vi "sutter_control2.vi"() -> ()   [LabVIEW 2014]
uses:
  <vilib>/Instr/_visa.llb/VISA Configure Serial Port (Instr).vi
panel:
  in  "下拉列表":u16(ring) items=["M1"=1, "M2"=2, "M3"=3, "M4"=4]
  in  "error in (no error)":errorcluster
  in  "Go Home":bool
  in  "stop":bool
  out "error out":errorcluster
  out "z-position":dbl
  out "y-position":dbl
  out "x-position":dbl
  in  "Z um":dbl
  in  "Y um":dbl
  in  "X um":dbl
  in  "VISA resource name":refnum<visa-resource-name>
  # "Back to (0 0 0)"
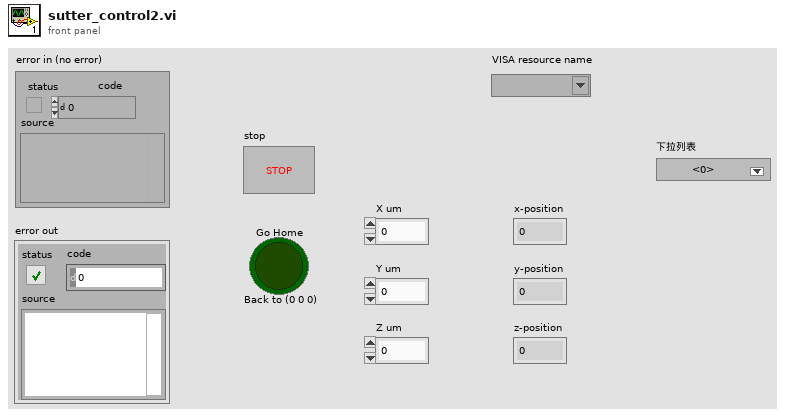
[diagram p1: front panel]
types:
  T1 = cluster{"Motor":u16, "X Pos":dbl, "Y Pos":dbl, "Z Pos":dbl, "Go Home":bool}
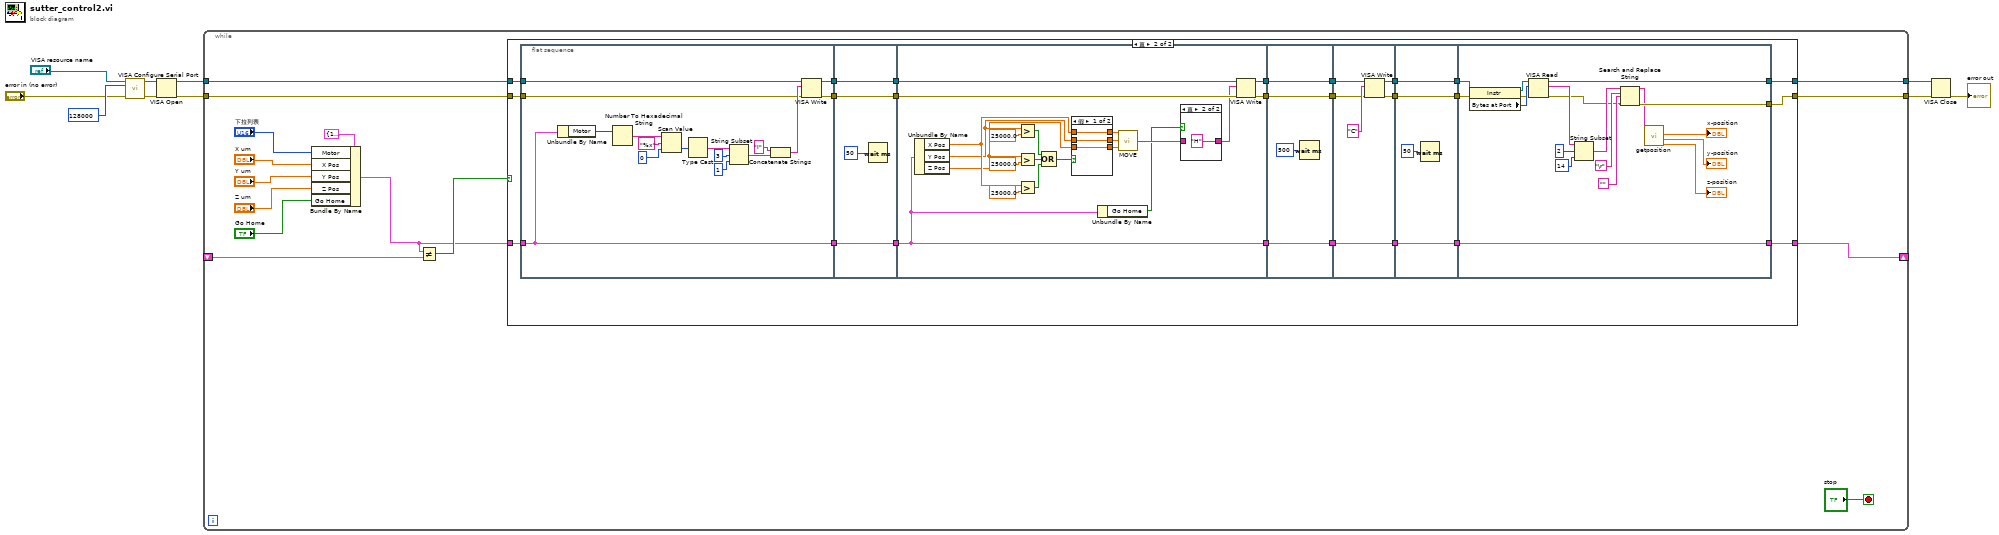
[diagram p0: block diagram]
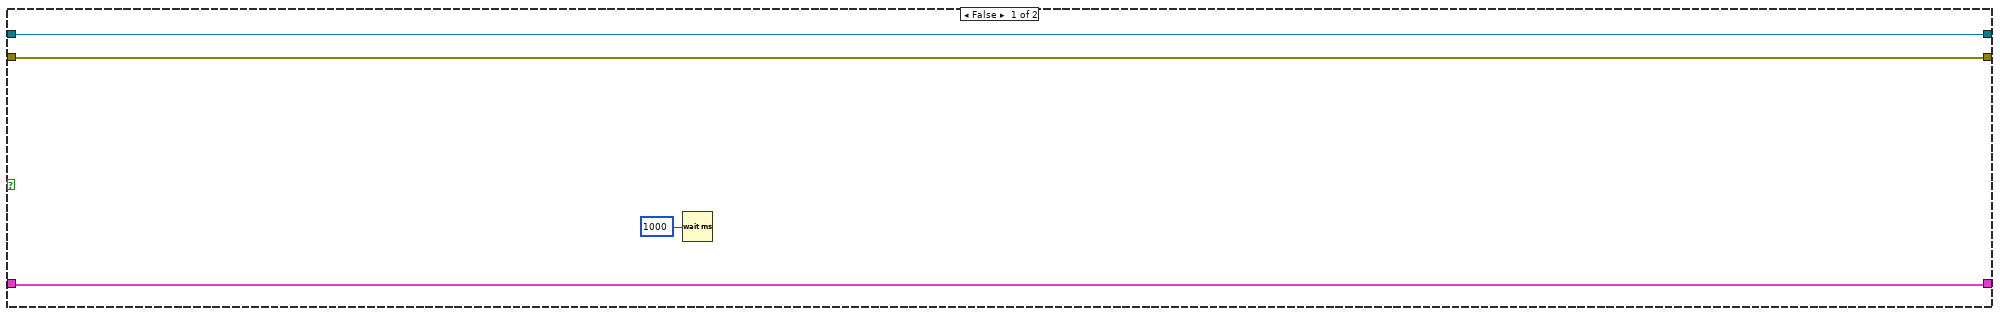
[diagram p2: hidden frame]
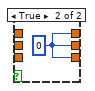
[diagram p4: hidden frame]
diagram:
  n1 = call-poly "VISA Configure Serial Port"("VISA resource name"="VISA resource name", "baud rate (9600)"=u32 128000, "error in (no error)"="error in (no error)") -> ("VISA resource name out"=w6:refnum<visa-resource-name>, "error out"=w2:errorcluster)  [unwired: 11 in]
  n2 = VISA Open(error in (no error)=w2, VISA resource name=w6) -> (VISA resource name=w5:refnum<visa-resource-name>, error out=w1:errorcluster)  [unwired: 3 in]
  n3 = while {
    tunnel: w1 -> [w22]
    tunnel: [w25] -> w7
    tunnel: w5 -> [w23]
    tunnel: [w21] -> w3
    shift-right: [w11] -> _
    shift-left: _ -> [w14]
    stop <- "stop" stop-if-true
    n4 = Bundle By Name(cluster=T1 {"Motor"=1, "X Pos"=0.0, "Y Pos"=0.0, "Z Pos"=0.0, "Go Home"=FALSE}, "Motor"="下拉列表", "X Pos"="X um", "Y Pos"="Y um", "Z Pos"="Z um", "Go Home"="Go Home") -> (w12:T1)
    n5 = Not Equal?(x=w12, y=w14) -> (x != y?=w13:bool)
    n6 = case shown="真" w13 {
      tunnel: [w26 w41] -> w25
      tunnel: w23 -> [w26 w40]
      tunnel: w22 -> [w27 w39]
      tunnel: [w27 w38] -> w21
      tunnel: w12 -> [w28 w37]
      tunnel: [w28 w30] -> w11
      frame False {
        n7 = Wait (ms)(milliseconds to wait=u32 1000 ("等待时间（毫秒）")) -> ()  [unwired: 1 out]
      }
      frame True {
        n8 = flat-sequence {
          tunnel: w39 -> [w57]
          tunnel: w40 -> [w69]
          tunnel: [w58] -> w53
          tunnel: [w56] -> w52
          tunnel: w37 -> [w54]
          tunnel: [w54] -> w31
          tunnel: [w73] -> w51
          tunnel: [w72] -> w50
          tunnel: w53 -> [w73]
          tunnel: w52 -> [w72]
          tunnel: [w70] -> w32
          tunnel: w31 -> [w70]
          tunnel: [w94] -> w49
          tunnel: [w93] -> w48
          tunnel: w51 -> [w92]
          tunnel: w50 -> [w91]
          tunnel: [w74] -> w33
          tunnel: w32 -> [w74]
          tunnel: w49 -> [w104]
          tunnel: [w104] -> w47
          tunnel: [w102] -> w46
          tunnel: w48 -> [w102]
          tunnel: [w101] -> w34
          tunnel: w33 -> [w101]
          tunnel: w47 -> [w107]
          tunnel: w46 -> [w109]
          tunnel: [w108] -> w45
          tunnel: [w106] -> w44
          tunnel: [w105] -> w35
          tunnel: w34 -> [w105]
          tunnel: w45 -> [w114]
          tunnel: [w114] -> w43
          tunnel: [w112] -> w42
          tunnel: w44 -> [w112]
          tunnel: [w111] -> w36
          tunnel: w35 -> [w111]
          tunnel: w43 -> [w128]
          tunnel: [w127] -> w41
          tunnel: w42 -> [w124]
          tunnel: [w122] -> w38
          tunnel: w36 -> [w115]
          tunnel: [w115] -> w30
          frame #0 {
            n9 = Unbundle By Name(w54) -> ("Motor"=w55:u16)
            n10 = Number To Hexadecimal String(2:w55) -> (0:w66:string)  [unwired: 1 in]
            n11 = Scan Value(string=w66, format string="%x", default (0 dbl)=0) -> (value=w64:i32)  [unwired: 1 out]
            n12 = Type Cast(x=w64) -> (*(type *) &x=w62:string)  [unwired: 1 in]
            n13 = String Subset(string=w62, offset (0)=3, length (rest)=1 ("length (rest)")) -> (substring=w59:string)
            n14 = Concatenate Strings("I" ("string"), w59) -> (w68:string)
            n15 = VISA Write(VISA resource name=w69, write buffer=w68, error in (no error)=w57) -> (VISA resource name out=w58:refnum<visa-resource-name>, error out=w56:errorcluster)  [unwired: 1 out]
          }
          frame #1 {
            n16 = Wait (ms)(milliseconds to wait=u32 50) -> ()  [unwired: 1 out]
          }
          frame #2 {
            n17 = Unbundle By Name(w74) -> ("X Pos"=w78:dbl, "Y Pos"=w77:dbl, "Z Pos"=w76:dbl)
            n18 = Greater?(x=w77, y=25000.0) -> (0:w87:bool)
            n19 = Greater?(x=w76, y=25000.0) -> (0:w86:bool)
            n20 = Greater?(x=w78, y=25000.0) -> (0:w85:bool)
            n21 = Compound Arithmetic op=OR(w87, w86, w85) -> (w84:bool)
            n22 = case shown="假" w84 {
              tunnel: [w99 w100] -> w83
              tunnel: w78 -> [w99 _]
              tunnel: [w98 w100] -> w82
              tunnel: w77 -> [w98 _]
              tunnel: [w97 w100] -> w81
              tunnel: w76 -> [w97 _]
              frame False {
              }
              frame True {
                w100 = 0
              }
            }
            n23 = Unbundle By Name(w74) -> ("Go Home"=w75:bool)
            n24 = call "MOVE.vi"("Z"=w81, "Y"=w82, "x"=w83) -> ("MOVE COMMAND"=w79:string)
            n25 = case shown="真" w75 {
              tunnel: [w95 "H" ("MOVE COMMAND")] -> w80
              tunnel: w79 -> [w95 _]
              frame False {
              }
              frame True {
              }
            }
            n26 = VISA Write(VISA resource name=w92, write buffer=w80, error in (no error)=w91) -> (VISA resource name out=w93:refnum<visa-resource-name>, error out=w94:errorcluster)  [unwired: 1 out]
          }
          frame #3 {
            n27 = Wait (ms)(milliseconds to wait=u32 500) -> ()  [unwired: 1 out]
          }
          frame #4 {
            n28 = VISA Write(VISA resource name=w109, write buffer="C", error in (no error)=w107) -> (VISA resource name out=w108:refnum<visa-resource-name>, error out=w106:errorcluster)  [unwired: 1 out]
          }
          frame #5 {
            n29 = Wait (ms)(milliseconds to wait=u32 50) -> ()  [unwired: 1 out]
          }
          frame #6 {
            n30 = property class="Instr"(reference=w128, error in=w124) -> (reference out=w133:refnum<visa-resource-name>, error out=w123:errorcluster, "Bytes at Port"=w129:u32)
            n31 = VISA Read(VISA resource name=w133, byte count=w129, error in (no error)=w123) -> (VISA resource name out=w127:refnum<visa-resource-name>, read buffer=w120:string, error out=w116:errorcluster)  [unwired: 1 out]
            n32 = String Subset(string=w120, offset (0)=2, length (rest)=14 ("length (rest)")) -> (substring=w117:string)
            n33 = Search and Replace String(input string=w117, search string="\r", replace string="", error in=w116) -> (result string=w121:string, error out=w122:errorcluster)  [unwired: 4 in, 2 out]
            n34 = call "getposition.vi"("string"=w121) -> ("x-position"=→"x-position":dbl, "y-position"=→"y-position":dbl, "z-position"=→"z-position":dbl)  [unwired: 1 out]
          }
        }
      }
    }
  }
  n35 = VISA Close(VISA resource name=w7, error in (no error)=w3) -> (error out=→"error out":errorcluster)
